vi "Make Test CAse.vi"(8 "error in (no error)":errorcluster) -> (0 "error out":errorcluster, 3 "LUnit Test Suite V2 out":refnum<class "LUnit Test Suite.lvclass">)   [LabVIEW 2020, in "Test Runner Test.lvclass"]
uses:
  Test Runner Test.lvclass
  source/API/LUnit Test Suite/LUnit Test Suite.lvclass
  Test Case Test Double Child/Light Test Case Double.lvclass
  C:/git/astemes-lunit/source/Core/LUnit Test Case/LUnit Test Case.lvclass
  Test Runner Test.lvclass/Test Runner Test.ctl
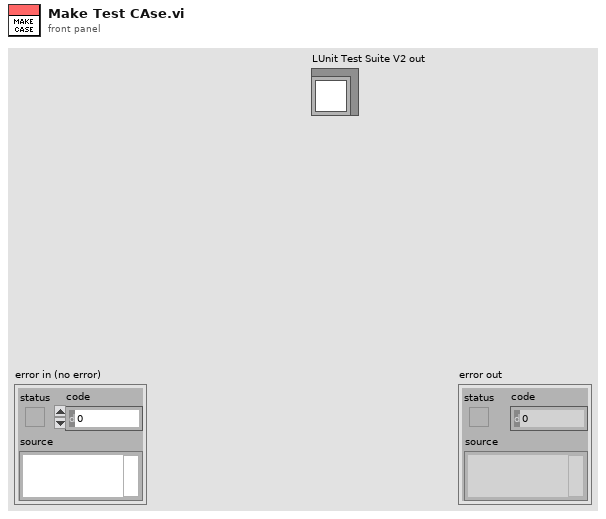
[diagram p1: front panel]
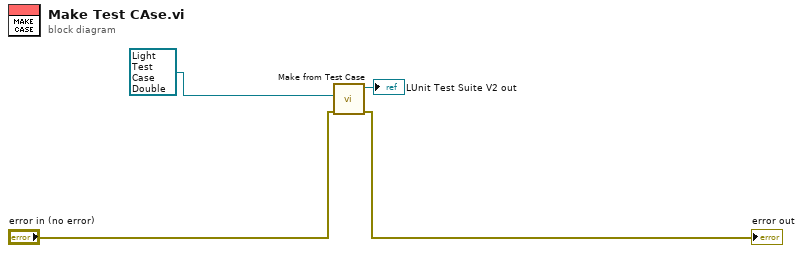
[diagram p0: block diagram]
diagram:
  n1 = call "Make from Test Case.vi"("error in (no error)"="error in (no error)", "LUnit Test Case"=refnum<class "Light Test Case Double.lvclass"> refnum ("Light Test Case Double.lvclass")) -> ("error out"=→"error out":errorcluster, "LUnit Test Suite Out"=→"LUnit Test Suite V2 out":refnum<class "LUnit Test Suite.lvclass">)  [unwired: 8 in]
